vi "各种状态子VI.vi"(2 "颜色输入":u32[](array[colorbox]), 3 "状态输入":string[][](array[string]), 4 "几种类型":i32=4, 5 "数值":u8) -> (0 "颜色":u32[](array[colorbox]), 1 "状态":string[](array[string]))   [LabVIEW 2013]
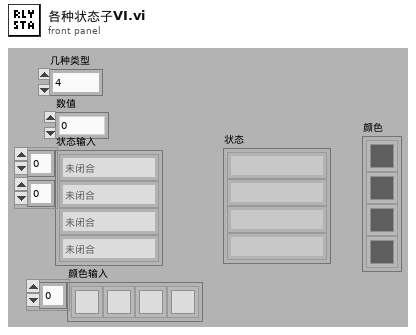
[diagram p1: front panel]
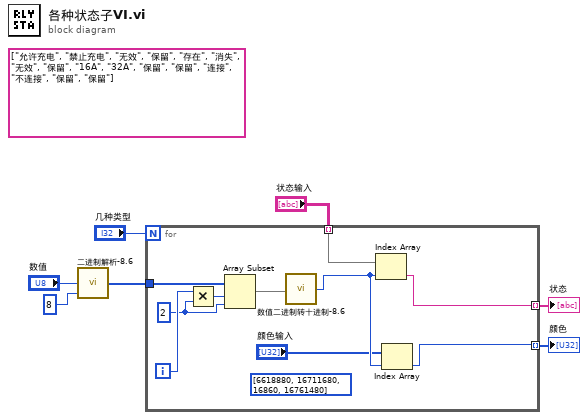
[diagram p0: block diagram]
diagram:
  (unwired) string[][] [["允许充电", "禁止充电", "无效", "保留"], ["存在", "消失", "无效", "保留"], ["16A", "32A", "保留", "保留"], ["连接", "不连接", "保留", "保留"]] ("状态输入")
  n1 = call "二进制解析-8.6.vi"("索引"=8, "数值"="数值") -> ("低位子数组"=w6:i32[])  [unwired: 3 out]
  n2 = for {
    N: "几种类型" -> [_]
    tunnel: w6 -> [w17]
    tunnel: [w12] -> w3 mode=indexing
    tunnel: [w10] -> w2 mode=indexing
    tunnel: "状态输入" -> [w9] mode=indexing
    i -> [w14]
    (unwired) u32[] [6618880, 16711680, 16860, 16761480]
    w13 = 2 ("y")
    n3 = Multiply(x=w14, y=w13) -> (x*y=w15:i32)
    n4 = Array Subset(array=w17, index=w15, length=w13) -> (w16:i32[])
    n5 = call "数值二进制转十进制-8.6.vi"("子数组"=w16) -> ("十进制数值"=w11:i32)  [unwired: 4 out]
    n6 = Index Array(array=w9, index=w11) -> (element=w12:string)
    n7 = Index Array(array="颜色输入", index=w11) -> (element=w10:u32)
  }
  "状态" <- w3
  "颜色" <- w2
